vi "Destroy.vi"(8 "error in (no error)":errorcluster, 11 "Event Registration Refnum":refnum<event-registration>) -> (0 "error out":errorcluster)   [LabVIEW 2017, in "WebServiceImporter.lvlib" / "Main Panel.lvlib" / "Preview.lvlib" / "Events.lvlib"]
uses:
  <vilib>/Platform/WebService/Main Panel/Pages/Preview/Events/Events.lvlib
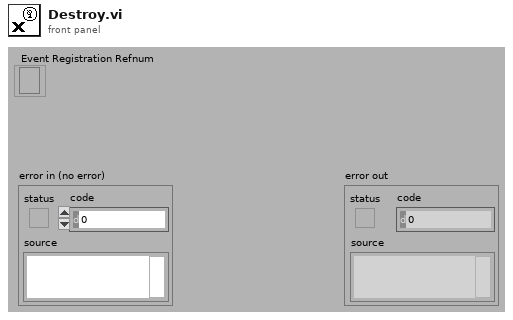
[diagram p1: front panel]
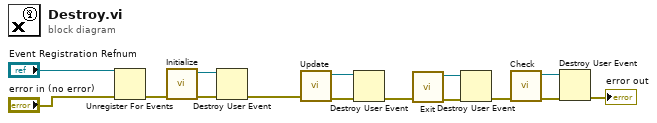
[diagram p0: block diagram]
diagram:
  n1 = Unregister For Events(event registration refnum="Event Registration Refnum", error in="error in (no error)") -> (error out=w11:errorcluster)
  n2 = call <vilib>:"Initialize.vi"("error in (no error)"=w11) -> ("error out"=w10:errorcluster, "user event (out)"=w14:refnum<user-event>)  [unwired: 9 in]
  n3 = Destroy User Event(user event=w14, error in=w10) -> (error out=w1:errorcluster)
  n4 = call <vilib>:"Update.vi"("error in (no error)"=w1) -> ("error out"=w3:errorcluster, "user event (out)"=w4:refnum<user-event>)  [unwired: 9 in]
  n5 = Destroy User Event(user event=w4, error in=w3) -> (error out=w2:errorcluster)
  n6 = call <vilib>:"Exit.vi"("error in (no error)"=w2) -> ("error out"=w5:errorcluster, "user event (out)"=w6:refnum<user-event>)  [unwired: 9 in]
  n7 = Destroy User Event(user event=w6, error in=w5) -> (error out=w7:errorcluster)
  n8 = call <vilib>:"Check.vi"("error in (no error)"=w7) -> ("error out"=w8:errorcluster, "user event (out)"=w9:refnum<user-event>)  [unwired: 9 in]
  n9 = Destroy User Event(user event=w9, error in=w8) -> (error out=→"error out":errorcluster)
